vi "WPI_MXP I2C Bus to first MXP Pin.vi"(7 "I2C Bus":T1) -> (8 "Shared MXP Pin":T2=enum."Invalid")   [LabVIEW 2017]
uses:
  <vilib>/Rock Robotics/WPI/MXP/WPI_MXP Shared MXP Pin.ctl
  <vilib>/Rock Robotics/SystemInterfaces/i2clib/i2c_bus.ctl
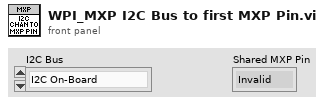
[diagram p1: front panel]
types:
  T1 = typedef "i2c_bus.ctl" = enum16{"I2C On-Board", "I2C MXP", "Invalid"}
  T2 = typedef "WPI_MXP Shared MXP Pin.ctl" = enum16{"11", "13", "15", "17", "19", "21", "23", "25", "27", "29", "31", "18", "22", "26", "32", "34", "Invalid"}
  T3 = enum16{"11", "13", "15", "17", "19", "21", "23", "25", "27", "29", "31", "18", "22", "26", "32", "34", "Invalid"}
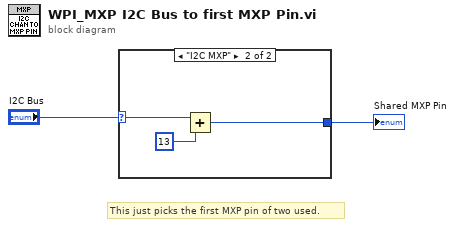
[diagram p0: block diagram]
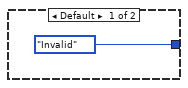
[diagram p2: hidden frame]
diagram:
  # "This just picks the first MXP pin of two used."
  n1 = case shown="\"I2C MXP\"" "I2C Bus" {
    selector: "I2C Bus" -> [_ w6]
    tunnel: [T3."Invalid" ("Shared MXP Pin") w5] -> w1
    frame Default {
    }
    frame "I2C MXP" {
      n2 = Add(x=w6, y=u16 13) -> (x+y=w5:u16)
    }
  }
  "Shared MXP Pin" <- w1
